vi "RC_calibration_ver2.vi"(8 "error in (no error)":errorcluster, 10 "Motors IDs Found":u8[](array[numeric]), 11 "VISA resource name":refnum<visa-resource-name>) -> (0 "error out":errorcluster, 1 "Dynamixel Cycles":T1, 2 "output cluster":T2={"Main Dynamixel Set Data"={"Lower Winch Bound (deg)"=0.0, "Upper Winch Bound (deg)"=1000.0}, "Rudder Dynamixel Set Data"={"Lower Winch Bound (deg)"=30.0, "Upper Winch Bound (deg)"=90.0}, "Jib Dynamixel Set Data"={"Lower Winch Bound (deg)"=0.0, "Upper Winch Bound (deg)"=1000.0}}, 3 "VISA resource name out":refnum<visa-resource-name>)   [LabVIEW 2013]
doc: "Allows the user to set the maximum and minimum points for the sails and center the rudder. Necessary because the Dynamixels can't measure their position along the pulley system.\n\nTakes in the port the Dynamixels are plugged into and the indexes of the motors. Outputs the minimum and maximum points for all three motors and what cycle the motors are at when the code ends along with the port and any errors that occurred."
uses:
  Data/TypeDefs/MotorSetup.ctl
  Data/TypeDefs/DynamixelSetupInfo.ctl
  Data/TypeDefs/DynamixelCycleTracker.ctl
  <instrlib>/Dynamixel Motor/Dynamixel Motor.lvlib
panel:
  in  "Dynamixel Cycles Constant":T1
  in  "Rudder centered?":bool
  in  "Rudder offset":dbl=30.0
  in  "Set Rudder position":dbl=150.0
  out "Rudder position":dbl
  in  "Jib movement 2":dbl
  out "Jib offset from\nmin to max":dbl
  out "Jib position\nat max":dbl
  out "Jib rotations to max":i32
  in  "Jib at maximum?":bool
  out "Jib minimum":dbl
  in  "Jib at minimum?":bool
  in  "Jib movement 1":dbl
  in  "Main movement 2":dbl
  out "Main offset from\nmin to max":dbl
  out "Main position\nat max":dbl
  out "Main rotations to max":i32
  in  "Main at maximum?":bool
  out "Main minimum":dbl
  in  "Main at minimum?":bool
  in  "Main movement 1":dbl
  # "TODO: Check labels for main/jib are right"
  # "1. Arrow up/down on main movement 1\n     to have sails move toward all in\n2. When it is as far in as is safe (given \n    pulleys) hit \"Main at minimum\" button"
  # "3. Arrow up/down on main movement 2 \n    to have sails move toward all out\n4. When it is as far out as is safe (given \n    pulleys) hit \"Main at maximum\" button"
  # "5. Arrow up/down on jib movement 1\n     to have sails move toward all in\n6. When it is as far in as is safe (given\n    pulleys) hit \"Jib at minimum\" button"
  # "7. Arrow up/down on jib movement 2 \n    to have sails move toward all out\n8. When it is as far out as is safe (given\n    pulleys) hit \"Jib at maximum\" button"
  # "9. Change rudder position until it is centered,\n     then hit \"rudder centered\"\n10. Set the offset from rudder center to min/max"
  # "Inputs/outputs you don't need to worry about"
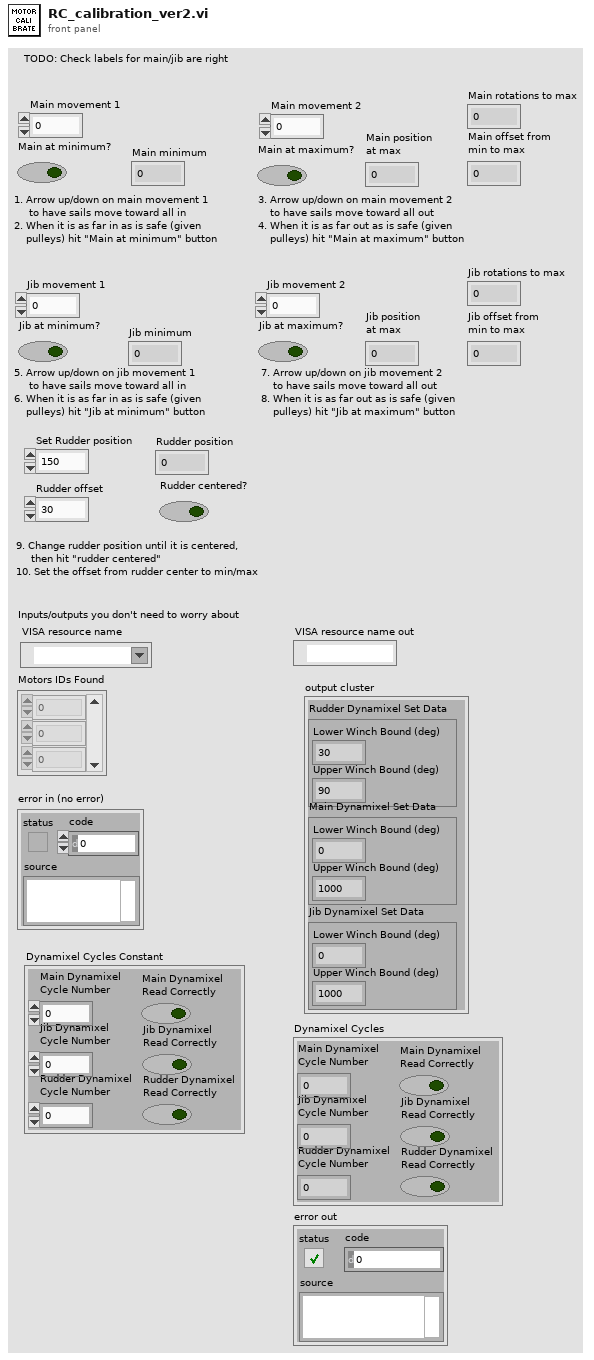
[diagram p1: front panel]
types:
  T1 = typedef "DynamixelCycleTracker.ctl" = cluster{"Main Dynamixel\nCycle Number":i32, "Jib Dynamixel\nCycle Number":i32, "Rudder Dynamixel\nCycle Number":i32, "Main Dynamixel\nRead Correctly":bool, "Jib Dynamixel\nRead Correctly":bool, "Rudder Dynamixel\nRead Correctly":bool}
  T2 = typedef "MotorSetup.ctl" = cluster{"Main Dynamixel Set Data":T3, "Rudder Dynamixel Set Data":T3, "Jib Dynamixel Set Data":T3}
  T3 = typedef "DynamixelSetupInfo.ctl" = cluster{"Lower Winch Bound (deg)":dbl, "Upper Winch Bound (deg)":dbl}
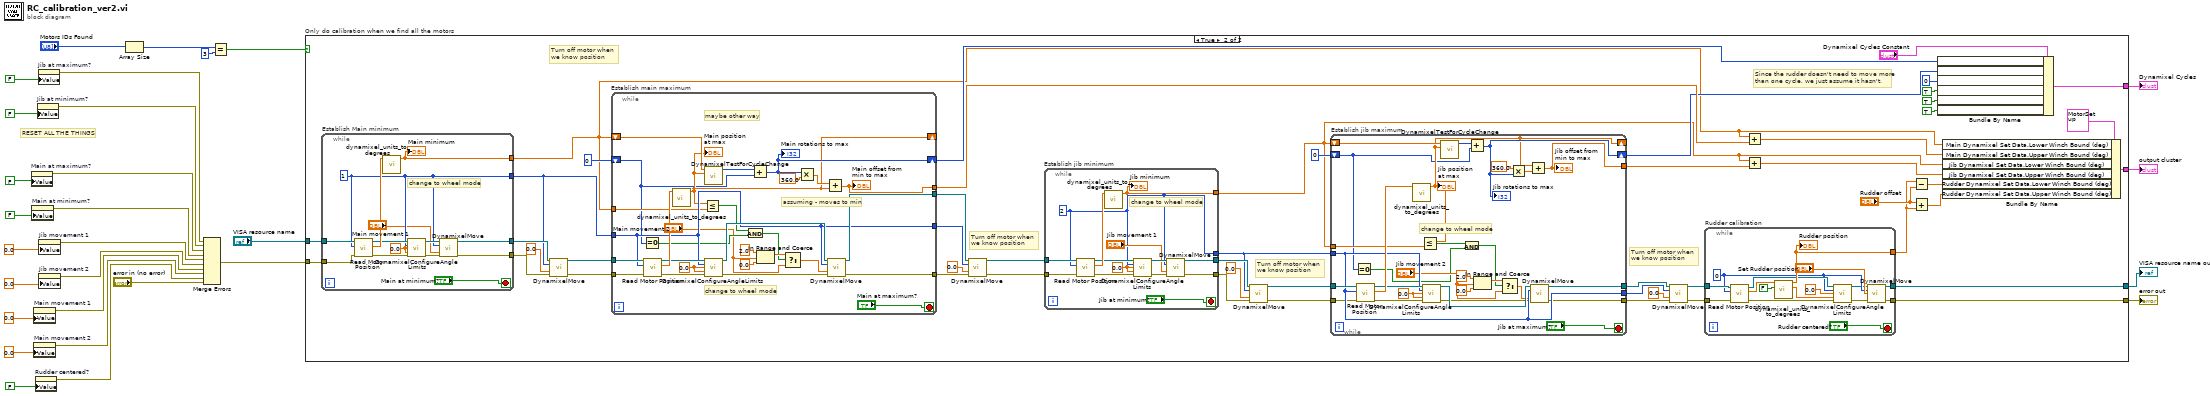
[diagram p0: block diagram]
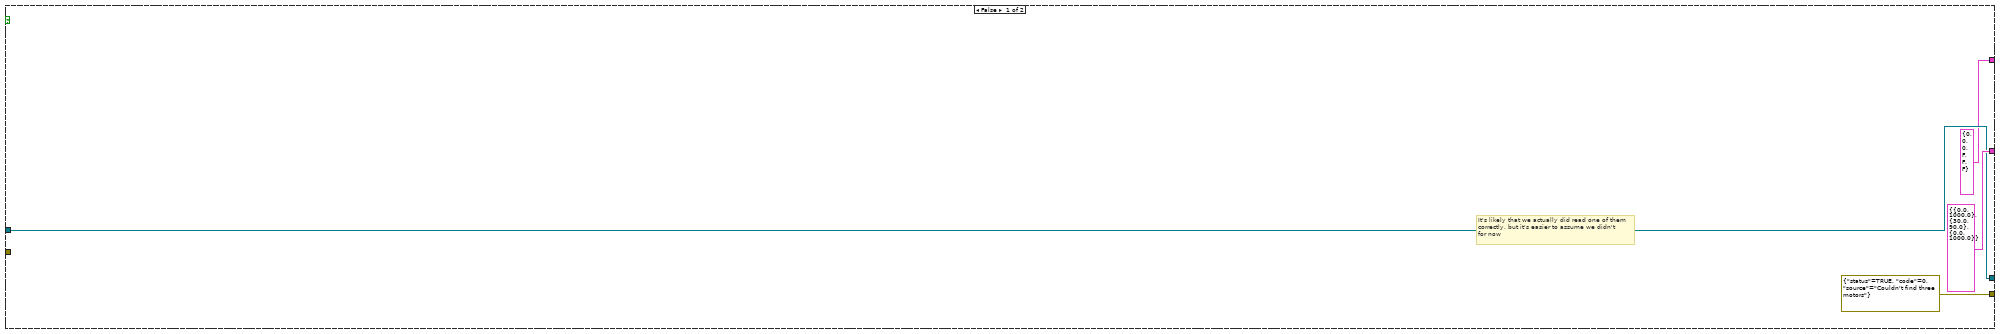
[diagram p2: hidden frame]
diagram:
  # "RESET ALL THE THINGS"
  n1 = property on="Main at maximum?" class="Bool (strict)"("Value"=FALSE ("Main at maximum?")) -> (error out=w3:errorcluster)  [unwired: 2 in, 1 out]
  n2 = property on="Main at minimum?" class="Bool (strict)"("Value"=FALSE ("Main at minimum?")) -> (error out=w4:errorcluster)  [unwired: 2 in, 1 out]
  n3 = property on="Main movement 1" class="DigNum (strict)"("Value"=0.0 ("Main movement 1")) -> (error out=w7:errorcluster)  [unwired: 2 in, 1 out]
  n4 = property on="Main movement 2" class="DigNum (strict)"("Value"=0.0 ("Main movement 2")) -> (error out=w8:errorcluster)  [unwired: 2 in, 1 out]
  n5 = property on="Rudder centered?" class="Bool (strict)"("Value"=FALSE ("Rudder centered?")) -> (error out=w9:errorcluster)  [unwired: 2 in, 1 out]
  n6 = property on="Jib at minimum?" class="Bool (strict)"("Value"=FALSE ("Jib at minimum?")) -> (error out=w2:errorcluster)  [unwired: 2 in, 1 out]
  n7 = property on="Jib at maximum?" class="Bool (strict)"("Value"=FALSE ("Jib at maximum?")) -> (error out=w1:errorcluster)  [unwired: 2 in, 1 out]
  n8 = property on="Jib movement 1" class="DigNum (strict)"("Value"=0.0 ("Jib movement 1")) -> (error out=w5:errorcluster)  [unwired: 2 in, 1 out]
  n9 = property on="Jib movement 2" class="DigNum (strict)"("Value"=0.0 ("Jib movement 2")) -> (error out=w6:errorcluster)  [unwired: 2 in, 1 out]
  n10 = Array Size(array="Motors IDs Found") -> (size(s)=w27:i32)
  n11 = Merge Errors(w1, w2, w3, w4, w5, w6, w7, w8, w9, "error in (no error)") -> (w11:errorcluster)
  n12 = Equal?(x=w27, y=3) -> (x = y?=w17:bool)
  n13 = case "Only do calibration when we find all the motors" shown="True" w17 {
    tunnel: "VISA resource name" -> [w32 w83]
    tunnel: [T2 {"Main Dynamixel Set Data"={"Lower Winch Bound (deg)"=0.0, "Upper Winch Bound (deg)"=1000.0}, "Rudder Dynamixel Set Data"={"Lower Winch Bound (deg)"=30.0, "Upper Winch Bound (deg)"=90.0}, "Jib Dynamixel Set Data"={"Lower Winch Bound (deg)"=0.0, "Upper Winch Bound (deg)"=1000.0}} ("Dynamixel Bounds Control") w46] -> w28
    tunnel: [w32 w45] -> w24
    tunnel: w11 -> [_ w59]
    tunnel: [errorcluster {"status"=TRUE, "code"=0, "source"="Couldn't find three motors"} ("error out") w44] -> w23
    tunnel: [T1 {"Main Dynamixel\nCycle Number"=0, "Jib Dynamixel\nCycle Number"=0, "Rudder Dynamixel\nCycle Number"=0, "Main Dynamixel\nRead Correctly"=FALSE, "Jib Dynamixel\nRead Correctly"=FALSE, "Rudder Dynamixel\nRead Correctly"=FALSE} ("Dynamixel Cycles Constant") w42] -> w22
    frame False {
      # "It's likely that we actually did read one of them\ncorrectly, but it's easier to assume we didn't \nfor now"
    }
    frame True {
      # "Since the rudder doesn't need to move more\nthan one cycle, we just assume it hasn't."
      # "Turn off motor when \nwe know position"
      # "Turn off motor when \nwe know position"
      # "Turn off motor when \nwe know position"
      # "Turn off motor when \nwe know position"
      n14 = while "Establish Main minimum" {
        tunnel: w83 -> [w155]
        tunnel: [w153] -> w35
        tunnel: [w149] -> w82
        tunnel: [w148] -> w77
        tunnel: w59 -> [w147]
        tunnel: [w144] -> w58
        stop <- "Main at minimum?" stop-if-true
        w151 = 0.0 ("Clockwise Angle Limit (0 deg)")
        w148 = u8 1 ("Motor ID (0)")
        # "change to wheel mode"
        n15 = call <instrlib>:"Read Motor Position.vi"("error in (no error)"=w147, "Motor ID (0)"=w148, "VISA resource name"=w155) -> ("error out"=w146:errorcluster, "Position (deg)"=w154:dbl, "VISA resource name out"=w152:refnum<visa-resource-name>)  [unwired: 6 in]
        n16 = call "dynamixel_units_to_degrees.vi"("Dynamixel Input"=w154) -> ("Degrees"=w153:dbl)  [unwired: 9 in, 1 out]
        "Main minimum" <- w153
        n17 = call "DynamixelConfigureAngleLimits.vi"("VISA resource name"=w152, "Motor ID (0)"=w148, "Clockwise Angle Limit (0 deg)"=w151, "Counter-Clockwise Angle Limit (300 deg)"=w151, "error in (no error)"=w146) -> ("VISA resource name out"=w150:refnum<visa-resource-name>, "error out"=w145:errorcluster)  [unwired: 9 in]
        n18 = call "DynamixelMove.vi"("VISA resource name"=w150, "Motor ID (0)"=w148, "Goal Speed (RPM)"="Main movement 1", "error in (no error)"=w145) -> ("VISA resource name out"=w149:refnum<visa-resource-name>, "error out"=w144:errorcluster)  [unwired: 10 in]
      }
      n19 = call "DynamixelMove.vi"("VISA resource name"=w82, "Motor ID (0)"=w77, "Goal Speed (RPM)"=0.0, "error in (no error)"=w58) -> ("VISA resource name out"=w80:refnum<visa-resource-name>, "error out"=w57:errorcluster)  [unwired: 10 in]
      n20 = while "Establish main maximum" {
        tunnel: w80 -> [w185]
        tunnel: [w180] -> w78
        tunnel: w77 -> [w177]
        tunnel: [w177] -> w65
        tunnel: w57 -> [w176]
        tunnel: [w173] -> w56
        shift-right: [w159] -> _
        shift-left: w35 -> [w172]
        shift-right: [w168] -> w41
        shift-left: 0 ("Dynamixel Cycle Number") -> [w157]
        tunnel: [w169] -> w49
        tunnel: w35 -> [w160]
        stop <- "Main at maximum?" stop-if-true
        w182 = 0.0 ("Clockwise Angle Limit (0 deg)")
        # "maybe other way"
        # "assuming - moves to min"
        # "change to wheel mode"
        n21 = Equal To 0?(x=w157) -> (x = 0?=w167:bool)
        n22 = call <instrlib>:"Read Motor Position.vi"("error in (no error)"=w176, "Motor ID (0)"=w177, "VISA resource name"=w185) -> ("error out"=w175:errorcluster, "Position (deg)"=w184:dbl, "VISA resource name out"=w183:refnum<visa-resource-name>)  [unwired: 6 in]
        n23 = call "dynamixel_units_to_degrees.vi"("Dynamixel Input"=w184) -> ("Degrees"=w159:dbl)  [unwired: 9 in, 1 out]
        "Main position\nat max" <- w159
        n24 = Less Or Equal?(x=w159, y=w160) -> (x <= y?=w158:bool)
        n25 = call "DynamixelTestForCycleChange.vi"("New position (deg)"=w159, "Old position (deg)"=w172) -> ("Dynamixel Cycle Number"=w170:i32)  [unwired: 9 in]
        n26 = call "DynamixelConfigureAngleLimits.vi"("VISA resource name"=w183, "Motor ID (0)"=w177, "Clockwise Angle Limit (0 deg)"=w182, "Counter-Clockwise Angle Limit (300 deg)"=w182, "error in (no error)"=w175) -> ("VISA resource name out"=w181:refnum<visa-resource-name>, "error out"=w174:errorcluster)  [unwired: 9 in]
        n27 = And(x=w158, y=w167) -> (x .and. y?=w163:bool)
        n28 = Add(x=w170, y=w157) -> (x+y=w168:i32)
        "Main rotations to max" <- w168
        n29 = In Range and Coerce(upper limit=2.0, x="Main movement 2", lower limit=0.0) -> (coerced(x)=w166:dbl)  [unwired: 1 out]
        n30 = Select(t=w166, s=w163, f="Main movement 2") -> (s? t:f=w161:dbl)
        n31 = Multiply(x=w168, y=360.0) -> (x*y=w171:dbl)
        n32 = Add(x=w171, y=w159) -> (x+y=w169:dbl)
        "Main offset from\nmin to max" <- w169
        n33 = call "DynamixelMove.vi"("VISA resource name"=w181, "Motor ID (0)"=w177, "Goal Speed (RPM)"=w161, "error in (no error)"=w174) -> ("VISA resource name out"=w180:refnum<visa-resource-name>, "error out"=w173:errorcluster)  [unwired: 10 in]
      }
      n34 = call "DynamixelMove.vi"("VISA resource name"=w78, "Motor ID (0)"=w65, "Goal Speed (RPM)"=0.0, "error in (no error)"=w56) -> ("VISA resource name out"=w76:refnum<visa-resource-name>, "error out"=w55:errorcluster)  [unwired: 10 in]
      n35 = while "Establish jib minimum" {
        tunnel: w76 -> [w137]
        tunnel: [w135] -> w74
        tunnel: [w134] -> w34
        tunnel: [w133] -> w72
        tunnel: w55 -> [w132]
        tunnel: [w129] -> w54
        stop <- "Jib at minimum?" stop-if-true
        w139 = 0.0 ("Clockwise Angle Limit (0 deg)")
        w133 = u8 2 ("Motor ID (0)")
        # "change to wheel mode"
        n36 = call <instrlib>:"Read Motor Position.vi"("error in (no error)"=w132, "Motor ID (0)"=w133, "VISA resource name"=w137) -> ("error out"=w131:errorcluster, "Position (deg)"=w141:dbl, "VISA resource name out"=w140:refnum<visa-resource-name>)  [unwired: 6 in]
        n37 = call "dynamixel_units_to_degrees.vi"("Dynamixel Input"=w141) -> ("Degrees"=w134:dbl)  [unwired: 9 in, 1 out]
        "Jib minimum" <- w134
        n38 = call "DynamixelConfigureAngleLimits.vi"("VISA resource name"=w140, "Motor ID (0)"=w133, "Clockwise Angle Limit (0 deg)"=w139, "Counter-Clockwise Angle Limit (300 deg)"=w139, "error in (no error)"=w131) -> ("VISA resource name out"=w138:refnum<visa-resource-name>, "error out"=w130:errorcluster)  [unwired: 9 in]
        n39 = call "DynamixelMove.vi"("VISA resource name"=w138, "Motor ID (0)"=w133, "Goal Speed (RPM)"="Jib movement 1", "error in (no error)"=w130) -> ("VISA resource name out"=w135:refnum<visa-resource-name>, "error out"=w129:errorcluster)  [unwired: 10 in]
      }
      n40 = call "DynamixelMove.vi"("VISA resource name"=w74, "Motor ID (0)"=w72, "Goal Speed (RPM)"=0.0, "error in (no error)"=w54) -> ("VISA resource name out"=w73:refnum<visa-resource-name>, "error out"=w53:errorcluster)  [unwired: 10 in]
      n41 = while "Establish jib maximum" {
        tunnel: w73 -> [w122]
        tunnel: w72 -> [w120]
        tunnel: [w121] -> w70
        tunnel: [w120] -> w69
        tunnel: [w119] -> w60
        tunnel: w53 -> [w118]
        tunnel: [w115] -> w52
        shift-right: [w104] -> _
        shift-left: w34 -> [w114]
        shift-right: [w111] -> w40
        shift-left: 0 -> [w100]
        tunnel: w34 -> [w103]
        stop <- "Jib at maximum?" stop-if-true
        w126 = 0.0 ("Clockwise Angle Limit (0 deg)")
        # "change to wheel mode"
        n42 = Equal To 0?(x=w100) -> (x = 0?=w101:bool)
        n43 = call <instrlib>:"Read Motor Position.vi"("error in (no error)"=w118, "Motor ID (0)"=w120, "VISA resource name"=w122) -> ("error out"=w117:errorcluster, "Position (deg)"=w128:dbl, "VISA resource name out"=w127:refnum<visa-resource-name>)  [unwired: 6 in]
        n44 = call "dynamixel_units_to_degrees.vi"("Dynamixel Input"=w128) -> ("Degrees"=w104:dbl)  [unwired: 9 in, 1 out]
        "Jib position\nat max" <- w104
        n45 = Less Or Equal?(x=w104, y=w103) -> (x <= y?=w102:bool)
        n46 = call "DynamixelConfigureAngleLimits.vi"("VISA resource name"=w127, "Motor ID (0)"=w120, "Clockwise Angle Limit (0 deg)"=w126, "Counter-Clockwise Angle Limit (300 deg)"=w126, "error in (no error)"=w117) -> ("VISA resource name out"=w125:refnum<visa-resource-name>, "error out"=w116:errorcluster)  [unwired: 9 in]
        n47 = call "DynamixelTestForCycleChange.vi"("New position (deg)"=w104, "Old position (deg)"=w114) -> ("Dynamixel Cycle Number"=w113:i32)  [unwired: 9 in]
        n48 = And(x=w102, y=w101) -> (x .and. y?=w107:bool)
        n49 = Add(x=w113, y=w100) -> (x+y=w111:i32)
        "Jib rotations to max" <- w111
        n50 = In Range and Coerce(upper limit=2.0, x="Jib movement 2", lower limit=0.0) -> (coerced(x)=w110:dbl)  [unwired: 1 out]
        n51 = Select(t=w110, s=w107, f="Jib movement 2") -> (s? t:f=w105:dbl)
        n52 = Multiply(x=360.0 ("y"), y=w111) -> (x*y=w124:dbl)
        n53 = Add(x=w104, y=w124) -> (x+y=w119:dbl)
        "Jib offset from\nmin to max" <- w119
        n54 = call "DynamixelMove.vi"("VISA resource name"=w125, "Motor ID (0)"=w120, "Goal Speed (RPM)"=w105, "error in (no error)"=w116) -> ("VISA resource name out"=w121:refnum<visa-resource-name>, "error out"=w115:errorcluster)  [unwired: 10 in]
      }
      n55 = call "DynamixelMove.vi"("VISA resource name"=w70, "Motor ID (0)"=w69, "Goal Speed (RPM)"=0.0, "error in (no error)"=w52) -> ("VISA resource name out"=w64:refnum<visa-resource-name>, "error out"=w51:errorcluster)  [unwired: 10 in]
      n56 = while "Rudder calibration" {
        tunnel: w64 -> [w99]
        tunnel: [w95] -> w47
        tunnel: [w94] -> w45
        tunnel: w51 -> [w93]
        tunnel: [w92] -> w44
        stop <- "Rudder centered?" stop-if-true
        w88 = u8 0 ("Motor ID (0)")
        n57 = call <instrlib>:"Read Motor Position.vi"("error in (no error)"=w93, "Motor ID (0)"=w88, "VISA resource name"=w99) -> ("error out"=w86:errorcluster, "Position (deg)"=w98:dbl, "VISA resource name out"=w90:refnum<visa-resource-name>)  [unwired: 6 in]
        n58 = call "dynamixel_units_to_degrees.vi"("MX Motor? (T)"=FALSE, "Dynamixel Input"=w98) -> ("Dynamixel units/cycle"=w89:dbl, "Degrees"=w95:dbl)  [unwired: 8 in]
        "Rudder position" <- w95
        n59 = call "DynamixelConfigureAngleLimits.vi"("VISA resource name"=w90, "Motor ID (0)"=w88, "Clockwise Angle Limit (0 deg)"=0.0, "Counter-Clockwise Angle Limit (300 deg)"=w89, "error in (no error)"=w86) -> ("VISA resource name out"=w84:refnum<visa-resource-name>, "error out"=w85:errorcluster)  [unwired: 9 in]
        n60 = call "DynamixelMove.vi"("VISA resource name"=w84, "Motor ID (0)"=w88, "Goal Position (150 deg)"="Set Rudder position", "error in (no error)"=w85) -> ("VISA resource name out"=w94:refnum<visa-resource-name>, "error out"=w92:errorcluster)  [unwired: 10 in]
      }
      n61 = Add(x=w35, y=w49) -> (x+y=w66:dbl)
      n62 = Add(x=w34, y=w60) -> (x+y=w67:dbl)
      n63 = Subtract(x=w47, y="Rudder offset") -> (x-y=w63:dbl)
      n64 = Add(x="Rudder offset", y=w47) -> (x+y=w61:dbl)
      n65 = Bundle By Name(cluster="Dynamixel Cycles Constant", "Main Dynamixel\nCycle Number"=w41, "Jib Dynamixel\nCycle Number"=w40, "Rudder Dynamixel\nCycle Number"=0 ("Rudder Dynamixel\nCycle Number"), "Main Dynamixel\nRead Correctly"=TRUE ("Main Dynamixel\nRead Correctly"), "Jib Dynamixel\nRead Correctly"=TRUE ("Jib Dynamixel\nRead Correctly"), "Rudder Dynamixel\nRead Correctly"=TRUE ("Rudder Dynamixel\nRead Correctly")) -> (w42:T1)
      n66 = Bundle By Name(cluster=T2 {"Main Dynamixel Set Data"={"Lower Winch Bound (deg)"=122.55131964809384, "Upper Winch Bound (deg)"=922.5513196480938}, "Rudder Dynamixel Set Data"={"Lower Winch Bound (deg)"=15.0, "Upper Winch Bound (deg)"=60.0}, "Jib Dynamixel Set Data"={"Lower Winch Bound (deg)"=241.0557184750733, "Upper Winch Bound (deg)"=1041.0557184750733}} ("Dynamixel Bounds Control"), "Main Dynamixel Set Data.Lower Winch Bound (deg)"=w35, "Main Dynamixel Set Data.Upper Winch Bound (deg)"=w66, "Jib Dynamixel Set Data.Lower Winch Bound (deg)"=w34, "Jib Dynamixel Set Data.Upper Winch Bound (deg)"=w67, "Rudder Dynamixel Set Data.Lower Winch Bound (deg)"=w63, "Rudder Dynamixel Set Data.Upper Winch Bound (deg)"=w61) -> (w46:T2)
    }
  }
  "output cluster" <- w28
  "VISA resource name out" <- w24
  "error out" <- w23
  "Dynamixel Cycles" <- w22
